vi "Convert To Detected Objects TensorFlow.vi"(7 "ROI Descriptor":T1 {"Contours"."Type" items=["No Selection", "Point", "Line", "Rectangle", "Oval", "Polygon", "Freehand Region", "Annulus", "Unused2", "Unused3", "Broken Line", "Freehand Line", "Rotated Rectangle"]}, 8 "error in (no error)":errorcluster, 9 "Labels":T5[](array[typedef]), 10 "Output Data Array":T4[](array[typedef]), 11 "Image":T2) -> (0 "error out":errorcluster, 1 "Number of Objects":i32, 2 "Detected Objects":T3[](array[typedef]) {"Bounding Box"."y" format="%.2f"; "Bounding Box"."x" format="%.2f"}, 3 "Image (duplicate)":T2)   [LabVIEW 2020]
uses:
  <vilib>/vision/Deep Learning.llb/IMAQ DL Model Label.ctl
  <vilib>/vision/Deep Learning.llb/IMAQ DL Model Output Data.ctl
  <vilib>/vision/Image Controls.llb/IMAQ Image.ctl
  <vilib>/vision/Deep Learning.llb/IMAQ DL Model Objects.ctl
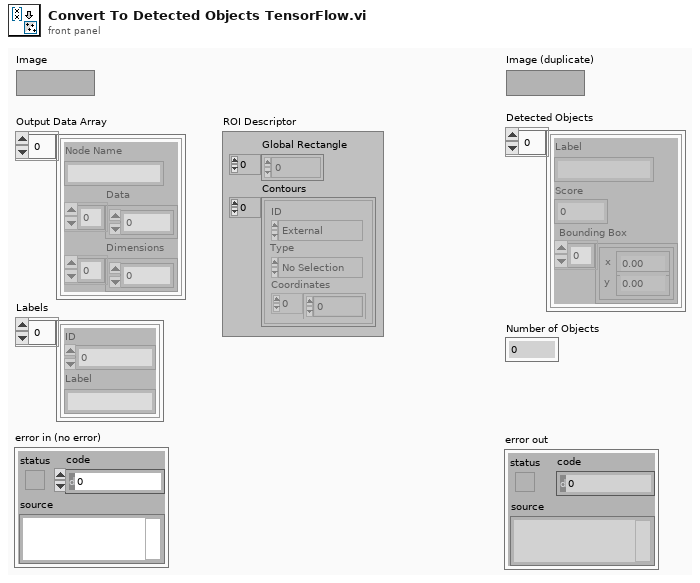
[diagram p1: front panel]
types:
  T1 = typedef "ROI Descriptor" = cluster{"Global Rectangle":i32[], "Contours":cluster{"ID":enum32{"External", "Internal"}, "Type":u32, "Coordinates":i32[]}[]}
  T2 = typedef "IMAQ Image.ctl" = refnum<image>
  T3 = typedef "IMAQ DL Model Objects.ctl" = cluster{"Label":string, "Score":sgl, "Bounding Box":cluster{"x":sgl, "y":sgl}[]}
  T4 = typedef "IMAQ DL Model Output Data.ctl" = cluster{"Node Name":string, "Data":sgl[], "Dimensions":u64[]}
  T5 = typedef "IMAQ DL Model Label.ctl" = cluster{"ID":u32, "Label":string}
  T6 = cluster{"Number of Objects":i32, "Labels":i32, "Scores":i32, "Bounding Boxes":i32}
  T7 = cluster{"t":cluster{i32, i32}, cluster{"X Resolution":i32, "Y Resolution":i32}}
  T8 = cluster{"t":cluster{sgl, sgl}, cluster{"X Resolution":sgl, "Y Resolution":sgl}}
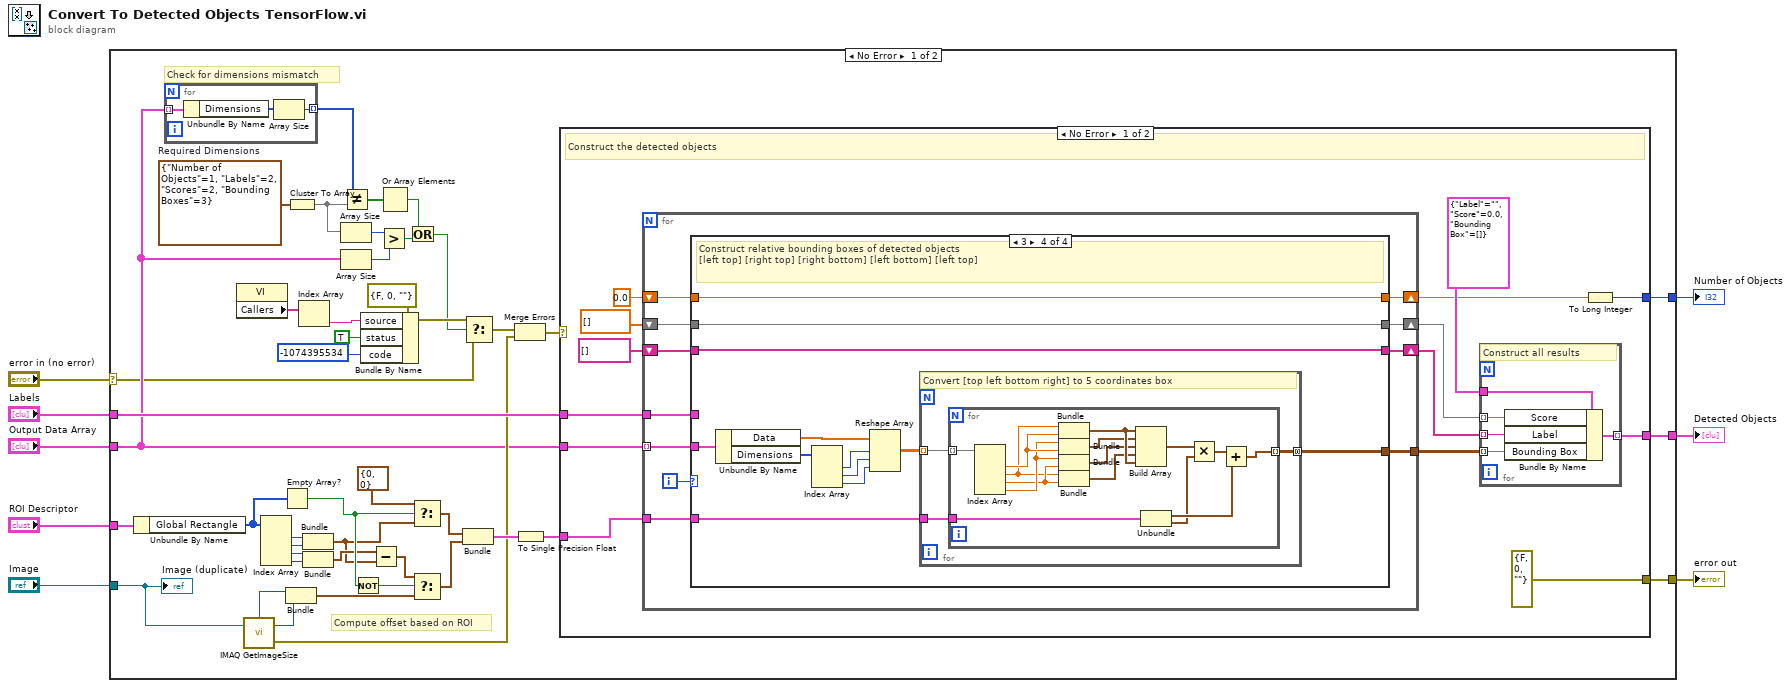
[diagram p0: block diagram]
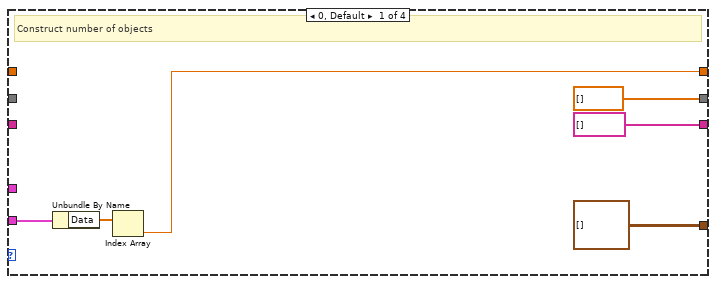
[diagram p2: hidden frame]
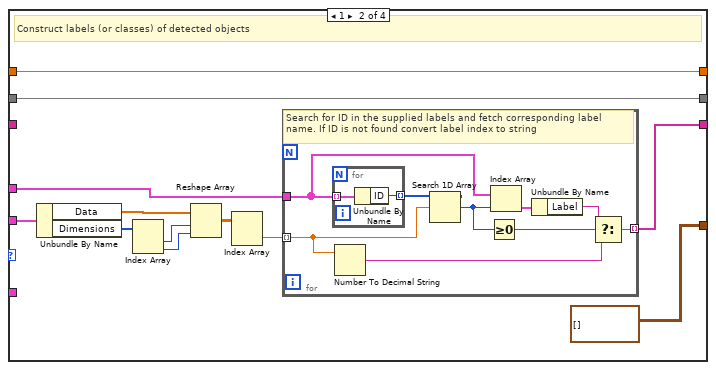
[diagram p3: hidden frame]
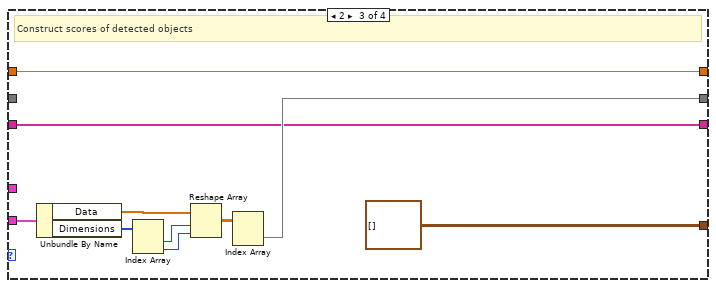
[diagram p4: hidden frame]
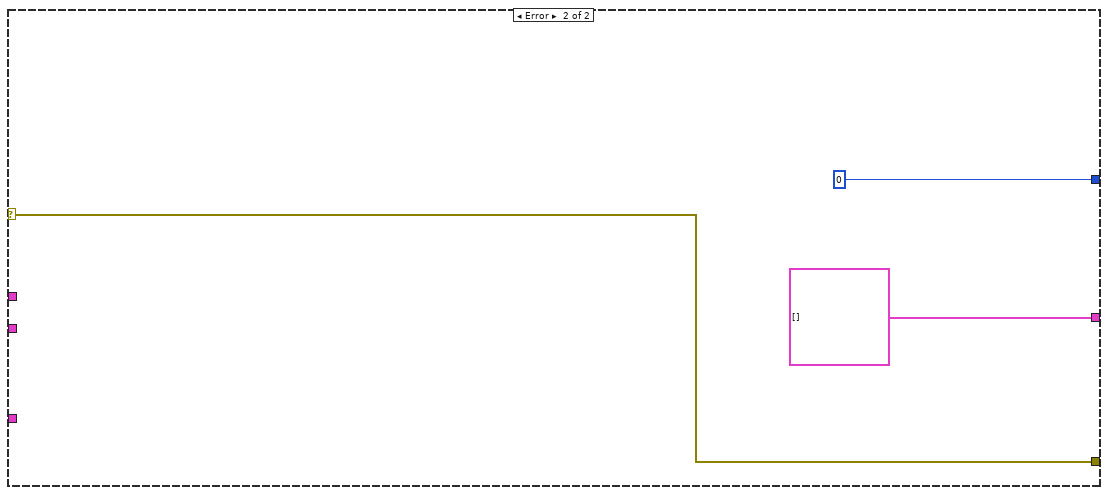
[diagram p5: hidden frame]
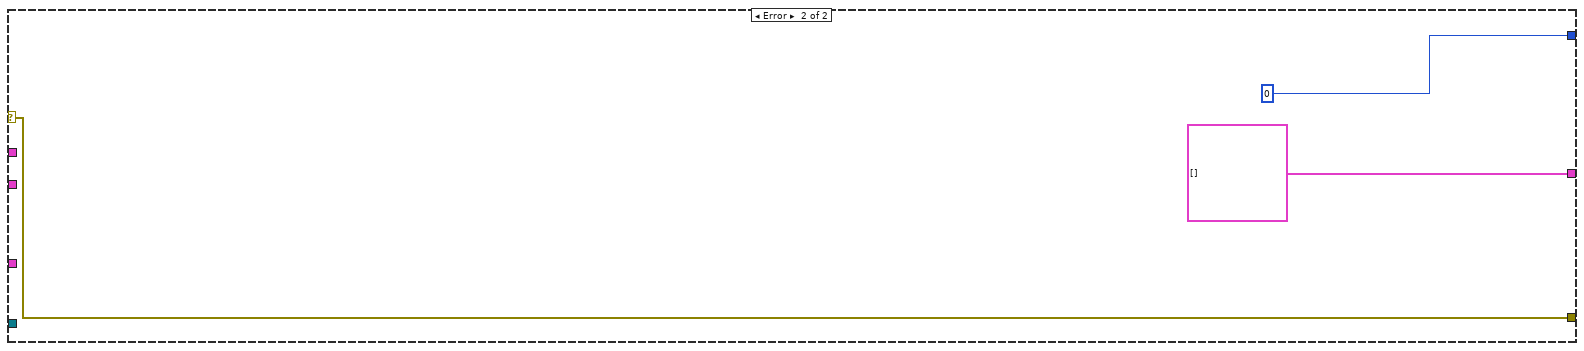
[diagram p6: hidden frame]
diagram:
  n1 = case shown="No Error" "error in (no error)" {
    selector: "error in (no error)" -> [w19 w158]
    tunnel: "Labels" -> [w49 _]
    tunnel: "Output Data Array" -> [w26 _]
    tunnel: [w47 w158] -> w5
    tunnel: [w48 T3[] []] -> w4
    tunnel: [w29 0] -> w3
    tunnel: "ROI Descriptor" -> [w46 _]
    tunnel: "Image" -> [w9 _]
    frame No Error {
      w43 = T6 {"Number of Objects"=1, "Labels"=2, "Scores"=2, "Bounding Boxes"=3}  # Required Dimensions
      # "Check for dimensions mismatch"
      # "Compute offset based on ROI"
      n2 = Unbundle By Name(w46) -> ("Global Rectangle"=w36:i32[])
      n3 = for {
        tunnel: w26 -> [w55] mode=indexing
        tunnel: [w53] -> w42 mode=indexing
        n4 = Unbundle By Name(w55) -> ("Dimensions"=w54:u64[])
        n5 = Array Size(array=w54) -> (size(s)=w53:i32)
      }
      n6 = property class="VI"() -> ("Callers"=w51:string[])  [unwired: 2 in, 2 out]
      n7 = call "IMAQ GetImageSize"("Image"=w9) -> ("Y Resolution"=w38:i32, "X Resolution"=w37:i32, "error out"=w32:errorcluster)  [unwired: 3 in]
      n8 = Index Array(array=w36) -> (element #1=w34:i32, element #2=w35:i32, element #3=w14:i32, element #4=w13:i32)  [unwired: 4 in]
      n9 = Empty Array?(array=w36) -> (empty?=w16:bool)
      n10 = Bundle("X Resolution"=w37, "Y Resolution"=w38) -> (w18:cluster{"X Resolution":i32, "Y Resolution":i32})  [unwired: 1 in]
      n11 = Cluster To Array(cluster=w43) -> (array=w25:i32[])
      n12 = Index Array(array=w51) -> (element=w50:string)  [unwired: 1 in]
      n13 = Bundle(w34, w35) -> (w11:cluster{i32, i32})  [unwired: 1 in]
      n14 = Bundle(w14, w13) -> (w12:cluster{i32, i32})  [unwired: 1 in]
      n15 = Array Size(array=w25) -> (size(s)=w24:i32)
      n16 = Array Size(array=w26) -> (size(s)=w23:i32)
      n17 = Not Equal?(x=w42, y=w25) -> (x != y?=w41:bool[])
      n18 = Not(x=w16) -> (.not. x?=w15:bool)
      n19 = Bundle By Name(cluster=errorcluster {"status"=FALSE, "code"=0, "source"=""} ("error in (no error)"), "source"=w50, "status"=TRUE, "code"=-1074395534) -> (w27:errorcluster)
      n20 = Subtract(x=w12, y=w11) -> (x-y=w10:cluster{i32, i32})
      n21 = Greater?(x=w24, y=w23) -> (0:w22:bool)
      n22 = Or Array Elements(Boolean array=w41) -> (logical OR=w21:bool)
      n23 = Or(x=w21, y=w22) -> (x .or. y?=w20:bool)
      n24 = Select(t=cluster{i32, i32} {0, 0}, s=w16, f=w11) -> (s? t:f=w30:cluster{i32, i32})
      n25 = Select(t=w10, s=w15, f=w18) -> (s? t:f=w17:cluster{"X Resolution":i32, "Y Resolution":i32})
      n26 = Bundle("t"=w30, w17) -> (w44:T7)  [unwired: 1 in]
      n27 = Select(t=w27, s=w20, f=w19) -> (s? t:f=w33:errorcluster)
      n28 = Merge Errors(w33, w32) -> (w45:errorcluster)
      n29 = To Single Precision Float(number=w44) -> (single precision float=w28:T8)
      n30 = case shown="No Error" w45 {
        selector: w45 -> [_ w157]
        tunnel: w26 -> [w69 _]
        tunnel: w49 -> [w66 _]
        tunnel: [w56 0] -> w29
        tunnel: [w61 T3[] []] -> w48
        tunnel: [errorcluster {"status"=FALSE, "code"=0, "source"=""} ("error IO") w157] -> w47
        tunnel: w28 -> [w59 _]
        frame No Error {
          # "Construct the detected objects"
          n31 = for {
            tunnel: w69 -> [w80] mode=indexing
            shift-right: [w78] -> w57
            shift-left: sgl 0.0 ("Numeric") -> [w77]
            shift-right: [w76] -> w64
            shift-left: sgl[] [] ("Data") -> [w75]
            tunnel: w66 -> [w74]
            shift-right: [w73] -> w63
            shift-left: string[] [] -> [w72]
            tunnel: [w71] -> w62
            tunnel: w59 -> [w70]
            i -> [w79]
            n32 = case shown="3" w79 {
              tunnel: w80 -> [w86 w93 w118 w125]
              tunnel: [w84 w97 w119 w129] -> w78
              tunnel: w77 -> [_ w97 w119 w129]
              tunnel: [sgl[] [] ("Data") w98 w112 w130] -> w76
              tunnel: w75 -> [_ w98 _ w130]
              tunnel: w74 -> [_ w90 _ _]
              tunnel: [string[] [] w87 w110 w131] -> w73
              tunnel: w72 -> [_ _ w110 w131]
              tunnel: [cluster{"Numeric":sgl, "Numeric":sgl}[][] [] cluster{"Numeric":sgl, "Numeric":sgl}[][] [] cluster{"Numeric":sgl, "Numeric":sgl}[][] [] w121] -> w71
              tunnel: w70 -> [_ _ _ w120]
              frame 0, Default {
                # "Construct number of objects"
                n33 = Unbundle By Name(w86) -> ("Data"=w85:sgl[])
                n34 = Index Array(array=w85) -> (element=w84:sgl)  [unwired: 1 in]
              }
              frame 1 {
                # "Construct labels (or classes) of detected objects"
                n35 = Unbundle By Name(w93) -> ("Data"=w91:sgl[], "Dimensions"=w92:u64[])
                n36 = Index Array(array=w92) -> (element #1=w96:u64, element #2=w88:u64)  [unwired: 2 in]
                n37 = Reshape Array(w91, w96, w88) -> (w95:sgl[][])
                n38 = Index Array(array=w95) -> (element=w94:sgl[])  [unwired: 2 in]
                n39 = for {
                  tunnel: w90 -> [w105]
                  tunnel: w94 -> [w103] mode=indexing
                  tunnel: [w99] -> w87 mode=indexing
                  # "Search for ID in the supplied labels and fetch corresponding label name. If ID is not found convert label index to string"
                  n40 = for {
                    tunnel: w105 -> [w109] mode=indexing
                    tunnel: [w108] -> w107 mode=indexing
                    n41 = Unbundle By Name(w109) -> ("ID"=w108:u32)
                  }
                  n42 = Number To Decimal String(number=w103) -> (decimal integer string=w100:string)  [unwired: 1 in]
                  n43 = Search 1D Array(1D array=w107, element=w103) -> (index of element=w106:i32)  [unwired: 1 in]
                  n44 = Greater Or Equal To 0?(x=w106) -> (x >= 0?=w102:bool)
                  n45 = Index Array(array=w105, index=w106) -> (element=w104:T5)
                  n46 = Unbundle By Name(w104) -> ("Label"=w101:string)
                  n47 = Select(t=w101, s=w102, f=w100) -> (s? t:f=w99:string)
                }
              }
              frame 2 {
                # "Construct scores of detected objects"
                n48 = Unbundle By Name(w118) -> ("Data"=w114:sgl[], "Dimensions"=w117:u64[])
                n49 = Index Array(array=w117) -> (element #1=w116:u64, element #2=w115:u64)  [unwired: 2 in]
                n50 = Reshape Array(w114, w116, w115) -> (w113:sgl[][])
                n51 = Index Array(array=w113) -> (element=w112:sgl[])  [unwired: 2 in]
              }
              frame 3 {
                # "Construct relative bounding boxes of detected objects\n[left top] [right top] [right bottom] [left bottom] [left top]"
                n52 = Unbundle By Name(w125) -> ("Data"=w126:sgl[], "Dimensions"=w127:u64[])
                n53 = Index Array(array=w127) -> (element #1=w128:u64, element #2=w124:u64, element #3=w123:u64)  [unwired: 3 in]
                n54 = Reshape Array(w126, w128, w124, w123) -> (w122:sgl[][][])
                n55 = for {
                  tunnel: [w134] -> w121 mode=concatenating
                  tunnel: w122 -> [w133] mode=indexing
                  tunnel: w120 -> [w132]
                  # "Convert [top left bottom right] to 5 coordinates box"
                  n56 = for {
                    tunnel: w133 -> [w136] mode=indexing
                    tunnel: [w145] -> w134 mode=indexing
                    tunnel: w132 -> [w149]
                    n57 = Index Array(array=w136) -> (element #1=w140:sgl, element #2=w137:sgl, element #3=w138:sgl, element #4=w139:sgl)  [unwired: 4 in]
                    n58 = Bundle("Numeric"=w137, "Numeric"=w140) -> (w144:cluster{"Numeric":sgl, "Numeric":sgl})  [unwired: 1 in]
                    n59 = Bundle("Numeric"=w139, "Numeric"=w140) -> (w142:cluster{"Numeric":sgl, "Numeric":sgl})  [unwired: 1 in]
                    n60 = Bundle("Numeric"=w139, "Numeric"=w138) -> (w143:cluster{"Numeric":sgl, "Numeric":sgl})  [unwired: 1 in]
                    n61 = Bundle("Numeric"=w137, "Numeric"=w138) -> (w141:cluster{"Numeric":sgl, "Numeric":sgl})  [unwired: 1 in]
                    n62 = Build Array(w144, w142, w143, w141, w144) -> (w135:cluster{"Numeric":sgl, "Numeric":sgl}[])
                    n63 = Unbundle(w149) -> ("t"=w148:cluster{sgl, sgl}, w146:cluster{"X Resolution":sgl, "Y Resolution":sgl})
                    n64 = Multiply(x=w135, y=w146) -> (x*y=w147:cluster{sgl, sgl}[])
                    n65 = Add(x=w147, y=w148) -> (x+y=w145:cluster{sgl, sgl}[])
                  }
                }
              }
            }
          }
          n66 = for {
            tunnel: T3 {"Label"="", "Score"=0.0, "Bounding Box"=[]} ("Class Result") -> [w154]
            tunnel: [w153] -> w61 mode=indexing
            tunnel: w64 -> [w152] mode=indexing
            tunnel: w63 -> [w151] mode=indexing
            tunnel: w62 -> [w150] mode=indexing
            # "Construct all results"
            n67 = Bundle By Name(cluster=w154, "Score"=w152, "Label"=w151, "Bounding Box"=w150) -> (w153:T3)
          }
          n68 = To Long Integer(number=w57) -> (32bit integer=w56:i32)
        }
        frame Error {
        }
      }
      "Image (duplicate)" <- w9
    }
    frame Error {
    }
  }
  "error out" <- w5
  "Detected Objects" <- w4
  "Number of Objects" <- w3
